vi "Update Tray Icon.vi"(0 "NotifyIcon in":refnum<class "NotifyIcon.lvclass">, 7 "Icon Reference":refnum<k24>, 11 "error in (no error)":errorcluster) -> (4 "NotifyIcon out":refnum<class "NotifyIcon.lvclass">, 15 "error out":errorcluster)   [LabVIEW 2016, in "NotifyIcon.lvclass"]
doc: "This VI assigns the input .NET Icon Class reference to the NotifyIcon Class.\n\n\nStinus Olsen\nCIM Industrial Systems A/S\n22. Feb. 2011 15:07\nmailto: seo@cim.as"
uses:
  NotifyIcon.lvclass
  System.Drawing
  NotifyIcon.lvclass/NotifyIcon.ctl
  System.Windows.Forms
panel:
  # "This VI belongs to the NotifyIcon Toolset. \nA toolset that makes it easy to create, control and manipulate a notification icon in the notification area of the Windows taskbar.\nThe toolset requires Microsoft .NET framework 2.0\n\n\nNOTICE -- YOU MUST LEAVE THIS NOTICE IN PLACE.  PER THE TERMS OF THE LICENSE BELOW, YOU MAY SUBLICENSE THIS SOFTWARE \nIN ANY WAY THAT DOES NOT CONFLICT WITH THIS LICENSE.\n\n### BSD License (http://www.opensource.org/licenses/bsd-license.php) Begin ###\n \nCopyright (c) 2011, Stinus Olsen <seo@cim.as>\n\nAll rights reserved.\n\nRedistribution and use in source and binary forms, with or without modification, are permitted provided that the following conditions are met:\n\n    * Redistributions of source code must retain the above copyright notice, this list of conditions and the following disclaimer.\n    * Redistributions in binary form must reproduce the above copyright notice, this list of conditions and the following disclaimer in the \n       documentation and/or other materials provided with the distribution.\n    * Neither the name of CIM Industrial Systems nor the names of its contributors may be used to endorse or promote products derived \n       from this software without specific prior written permission.\n\nTHIS SOFTWARE IS PROVIDED BY THE COPYRIGHT HOLDERS AND CONTRIBUTORS \"AS IS\" AND ANY EXPRESS OR IMPLIED WARRANTIES, \nINCLUDING, BUT NOT LIMITED TO, THE IMPLIED WARRANTIES OF MERCHANTABILITY AND FITNESS FOR A PARTICULAR PURPOSE ARE \nDISCLAIMED. IN NO EVENT SHALL THE COPYRIGHT OWNER OR CONTRIBUTORS BE LIABLE FOR ANY DIRECT, INDIRECT, INCIDENTAL,\n SPECIAL, EXEMPLARY, OR CONSEQUENTIAL DAMAGES (INCLUDING, BUT NOT LIMITED TO, PROCUREMENT OF SUBSTITUTE GOODS OR \nSERVICES; LOSS OF USE, DATA, OR PROFITS; OR BUSINESS INTERRUPTION) HOWEVER CAUSED AND ON ANY THEORY OF LIABILITY, \nWHETHER IN CONTRACT, STRICT LIABILITY, OR TORT (INCLUDING NEGLIGENCE OR OTHERWISE) ARISING IN ANY WAY OUT OF THE USE \nOF THIS SOFTWARE, EVEN IF ADVISED OF THE POSSIBILITY OF SUCH DAMAGE.\n\n### BSD License End ###"
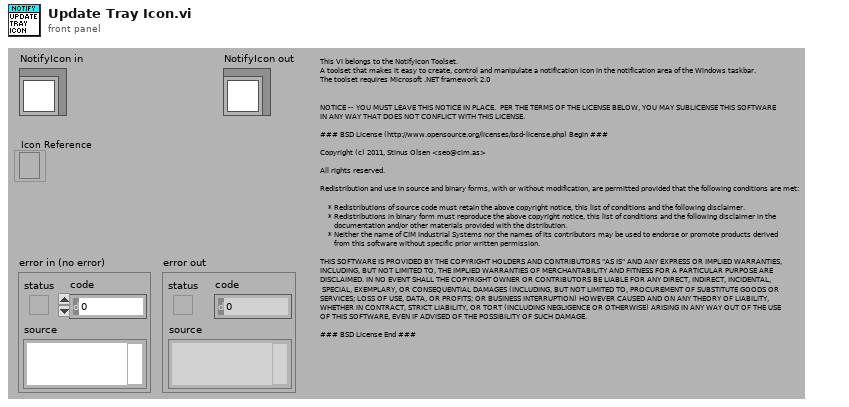
[diagram p1: front panel]
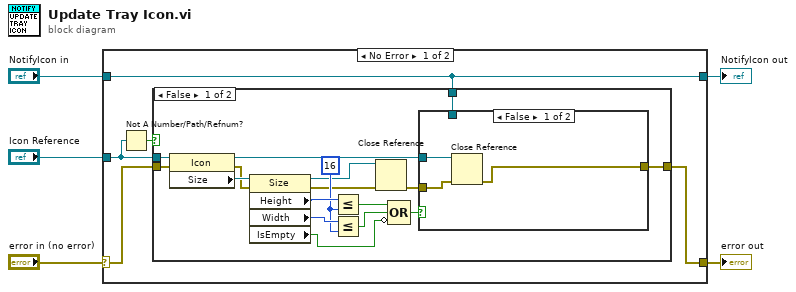
[diagram p0: block diagram]
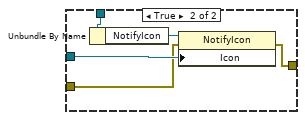
[diagram p2: hidden frame]
diagram:
  n1 = case shown="No Error" "error in (no error)" {
    selector: "error in (no error)" -> [w8 w38]
    tunnel: [w6 w38] -> w5
    tunnel: [w7 w37] -> w3
    tunnel: "NotifyIcon in" -> [w7 w37]
    tunnel: "Icon Reference" -> [w9 _]
    frame No Error {
      n2 = Not A Number/Path/Refnum?(number/path/refnum=w9) -> (NaN/Path/Refnum?=w10:bool)
      n3 = case shown="False" w10 {
        tunnel: w9 -> [w27 _]
        tunnel: w8 -> [w26 w36]
        tunnel: w7 -> [w17 _]
        tunnel: [w11 w36] -> w6
        frame False {
          w22 = 16 ("Int32 width")
          n4 = property class="Icon"(reference=w27, error in=w26) -> (reference out=w13:refnum<k24>, error out=w14:errorcluster, "Size"=w25:refnum<k24>)
          n5 = property class="Size"(reference=w25, error in=w14) -> (reference out=w16:refnum<k24>, error out=w15:errorcluster, "Height"=w24:i32, "Width"=w23:i32, "IsEmpty"=w19:bool)
          n6 = Less Or Equal?(x=w24, y=w22) -> (x <= y?=w21:bool)
          n7 = Less Or Equal?(x=w23, y=w22) -> (x <= y?=w20:bool)
          n8 = Close Reference(reference=w16, error in (no error)=w15) -> (error out=w12:errorcluster)
          n9 = Compound Arithmetic op=OR(w21, w20, invert w19) -> (w18:bool)
          n10 = case shown="False" w18 {
            tunnel: w17 -> [_ w34]
            tunnel: w13 -> [w30 w33]
            tunnel: w12 -> [w29 w32]
            tunnel: [w28 w31] -> w11
            frame False {
              n11 = Close Reference(reference=w30, error in (no error)=w29) -> (error out=w28:errorcluster)
            }
            frame True {
              n12 = Unbundle By Name(w34) -> ("NotifyIcon"=w35:refnum<k24>)
              n13 = property class="NotifyIcon"(reference=w35, error in=w32, "Icon"=w33) -> (error out=w31:errorcluster)  [unwired: 1 out]
            }
          }
        }
        frame True {
        }
      }
    }
    frame Error {
    }
  }
  "error out" <- w5
  "NotifyIcon out" <- w3
